vi "LogEvent.vi"(8 "error in (no error)":errorcluster, 9 "eventInfo":dbl=nan, 10 "Event Name":string="acquireFixation", 11 "TrialBasedExperiment in":refnum<class "MatlabExperiment.lvclass">) -> (0 "error out":errorcluster, 3 "TrialBasedExperiment out":refnum<class "MatlabExperiment.lvclass">)   [LabVIEW 2010, in "MatlabExperiment.lvclass"]
uses:
  MatlabExperiment.lvclass
  Core SubVIs/Core SubVIs.lvlib
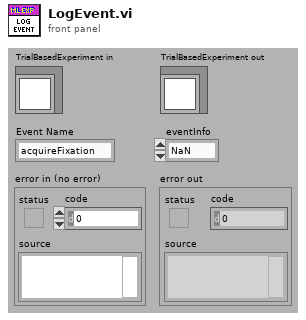
[diagram p1: front panel]
types:
  T1 = enum16{"Get Time", "Get Elapsed Time", "Reset Elapsed Time"}
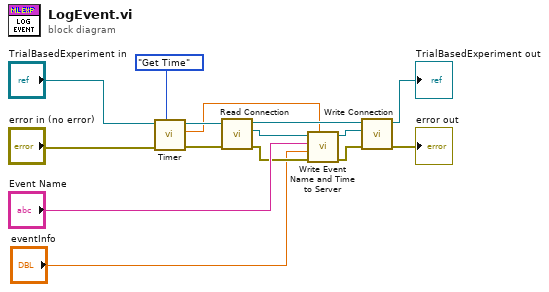
[diagram p0: block diagram]
diagram:
  n1 = call-dynamic "Timer.vi"("Method"=T1."Get Time", "error in (no error)"="error in (no error)", "BehaviorData in"="TrialBasedExperiment in") -> ("error out"=w6:errorcluster, "Time"=w1:dbl, "BehaviorData out"=w5:refnum<class "MatlabExperiment.lvclass">)  [unwired: 5 in, 1 out]
  n2 = call-dynamic "Read Connection.vi"("error in (no error)"=w6, "TrialBasedExperiment in"=w5) -> ("error out"=w9:errorcluster, "Connection"=w13:refnum<k5>, "TrialBasedExperiment out"=w11:refnum<class "MatlabExperiment.lvclass">)  [unwired: 7 in]
  n3 = call "Write Event Name and Time to Server.vi"("Timer Value (ms)"=w1, "error in (no error)"=w9, "eventInfo"="eventInfo", "Event Name"="Event Name", "connection ID"=w13) -> ("error out"=w8:errorcluster, "connection ID duplicate"=w12:refnum<k5>)  [unwired: 5 out]
  n4 = call-dynamic "Write Connection.vi"("error in (no error)"=w8, "Connection"=w12, "TrialBasedExperiment in"=w11) -> ("error out"=→"error out":errorcluster, "TrialBasedExperiment out"=→"TrialBasedExperiment out":refnum<class "MatlabExperiment.lvclass">)  [unwired: 7 in]
